vi "Asynchronous - Update RT to BC Data - Preprocess Map.vi"(8 "error in (no error)":errorcluster, 11 "Map (RT to BC)":T2[](array[typedef]) {"Word Data Reference" format="%.0x"}) -> (0 "error out":errorcluster, 3 "Frames":T1[](array[typedef]))   [LabVIEW 2017, in "Ballard MIL-1553 Engine.lvlib"]
uses:
  Ballard MIL-1553 Engine.lvlib
  Controls/RT Async_Map RT2BC.ctl
  <vilib>/NI Veristand/Custom Device API/Data Reference.ctl
  Controls/RT Async_Map_Type.ctl
  Controls/Asynchronous - Update RT to BC Data - Map.ctl
  <vilib>/NI VeriStand/Custom Device API/Custom Device API.lvlib
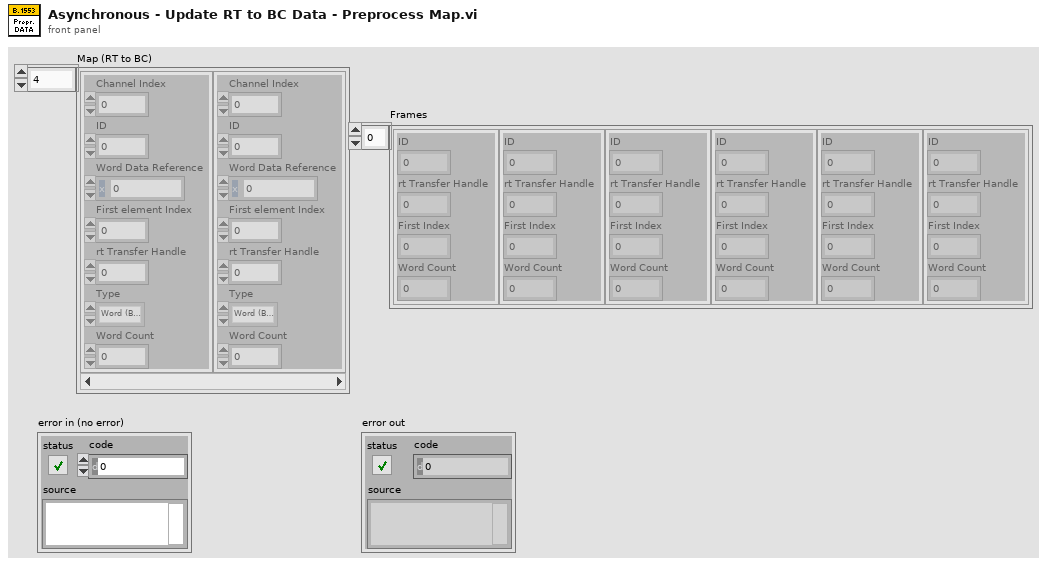
[diagram p1: front panel]
types:
  T1 = typedef "Ballard MIL-1553 Engine.lvlib/Asynchronous - Update RT to BC Data - Map.ctl" = cluster{"ID":i32, "rt Transfer Handle":u64, "First Index":i32, "Word Count":i32}
  T2 = typedef "Ballard MIL-1553 Engine.lvlib/RT Async_Map RT2BC.ctl" = cluster{"Channel Index":i32, "ID":i32, "Word Data Reference":T3, "First element Index":i32, "rt Transfer Handle":u64, "Type":T4, "Word Count":i32}
  T3 = typedef "Custom Device API.lvlib/Data Reference.ctl" = i32
  T4 = typedef "Ballard MIL-1553 Engine.lvlib/RT Async_Map_Type.ctl" = enum16{"Word (BC to RT)", "Word (MC (Rx))", "Acyclic Message Trigger", "Word (RT to ..)", "Word (RT to RT)", "Word (MC (Tx))", "RT Status", "BC Commands", "RT Commands"}
  T5 = cluster{"ID":i32, "rt Transfer Handle":u64, "Indexes":i32[]}[]
  T6 = cluster{"ID":i32, "rt Transfer Handle":u64, "Indexes":i32[]}
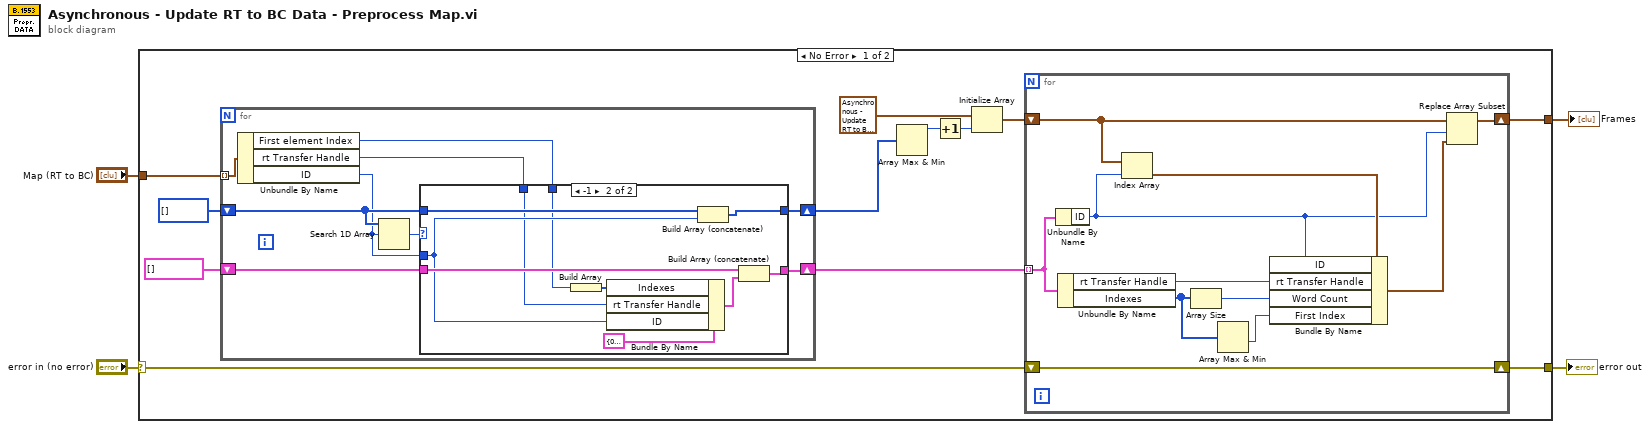
[diagram p0: block diagram]
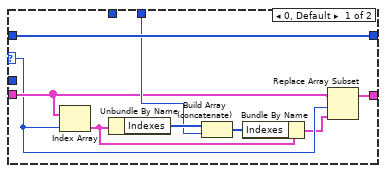
[diagram p2: hidden frame]
diagram:
  n1 = case shown="No Error" "error in (no error)" {
    selector: "error in (no error)" -> [w10 w56]
    tunnel: [w9 w56] -> w3
    tunnel: "Map (RT to BC)" -> [w16 _]
    tunnel: [w11 _] -> w1
    frame No Error {
      n2 = for {
        tunnel: w16 -> [w36] mode=indexing
        shift-right: [w29] -> w6
        shift-left: i32[] [] -> [w33]
        shift-right: [w28] -> w5
        shift-left: T5 [] -> [w34]
        n3 = Unbundle By Name(w36) -> ("First element Index"=w30:i32, "rt Transfer Handle"=w31:u64, "ID"=w32:i32)
        n4 = Search 1D Array(1D array=w33, element=w32) -> (index of element=w35:i32)  [unwired: 1 in]
        n5 = case shown="-1" w35 {
          selector: w35 -> [w41 _]
          tunnel: w34 -> [w42 w52]
          tunnel: w33 -> [w45 w55]
          tunnel: w32 -> [_ w49]
          tunnel: w31 -> [_ w48]
          tunnel: w30 -> [w43 w47]
          tunnel: [w45 w54] -> w29
          tunnel: [w37 w50] -> w28
          frame 0, Default {
            n6 = Index Array(array=w42, index=w41) -> (element=w40:T6)
            n7 = Unbundle By Name(w40) -> ("Indexes"=w44:i32[])
            n8 = Build Array (concatenate)(w44, w43) -> (w39:i32[])
            n9 = Bundle By Name(cluster=w40, "Indexes"=w39) -> (w38:T6)
            n10 = Replace Array Subset(array=w42, new element=w38, index=w41) -> (w37:T5)
          }
          frame -1 {
            n11 = Build Array(w47) -> (w46:i32[])
            n12 = Bundle By Name(cluster=T6 {"ID"=0, "rt Transfer Handle"=0, "Indexes"=[]}, "Indexes"=w46, "rt Transfer Handle"=w48, "ID"=w49) -> (w51:T6)
            n13 = Build Array (concatenate)(w55, w49) -> (w54:i32[])
            n14 = Build Array (concatenate)(w52, w51) -> (w50:T5)
          }
        }
      }
      n15 = Array Max & Min(array=w6) -> (max value=w15:i32)  [unwired: 3 out]
      n16 = Increment(x=w15) -> (x+1=w14:i32)
      n17 = Initialize Array(T1 {"ID"=-1, "rt Transfer Handle"=18446744073709551615, "First Index"=-1, "Word Count"=-1} ("Map Entry"), w14) -> (w12:T1[])
      n18 = for {
        shift-right: [w25] -> w11
        shift-left: w12 -> [w26]
        shift-right: [w27] -> w9
        shift-left: w10 -> [w27]
        tunnel: w5 -> [w21] mode=indexing
        n19 = Unbundle By Name(w21) -> ("ID"=w22:i32)
        n20 = Unbundle By Name(w21) -> ("rt Transfer Handle"=w20:u64, "Indexes"=w18:i32[])
        n21 = Index Array(array=w26, index=w22) -> (element=w24:T1)
        n22 = Array Size(array=w18) -> (size(s)=w19:i32)
        n23 = Array Max & Min(array=w18) -> (min value=w17:i32)  [unwired: 3 out]
        n24 = Bundle By Name(cluster=w24, "ID"=w22, "rt Transfer Handle"=w20, "Word Count"=w19, "First Index"=w17) -> (w23:T1)
        n25 = Replace Array Subset(array=w26, new element=w23, index=w22) -> (w25:T1[])
      }
    }
    frame Error {
    }
  }
  "error out" <- w3
  "Frames" <- w1
